vi "clientTCP.vi"(3 "error in":errorcluster, 5 "BrigthField":T1(plugin-control)) -> (0 "error out":errorcluster, 1 "maskCenters":u32[][](array[numeric]), 2 "Segmented":T1(plugin-control))   [LabVIEW 2018]
uses:
  <resource>/objmgr/IMAQImage.rc
panel:
  out "call chain":string[](array[string])
  out "ySize 2":i32
  out "xSize 2":i32
  out "Image 3":T1(plugin-control)
  out "ySize":i32
  out "xSize":i32
  in  "Image File Path":path
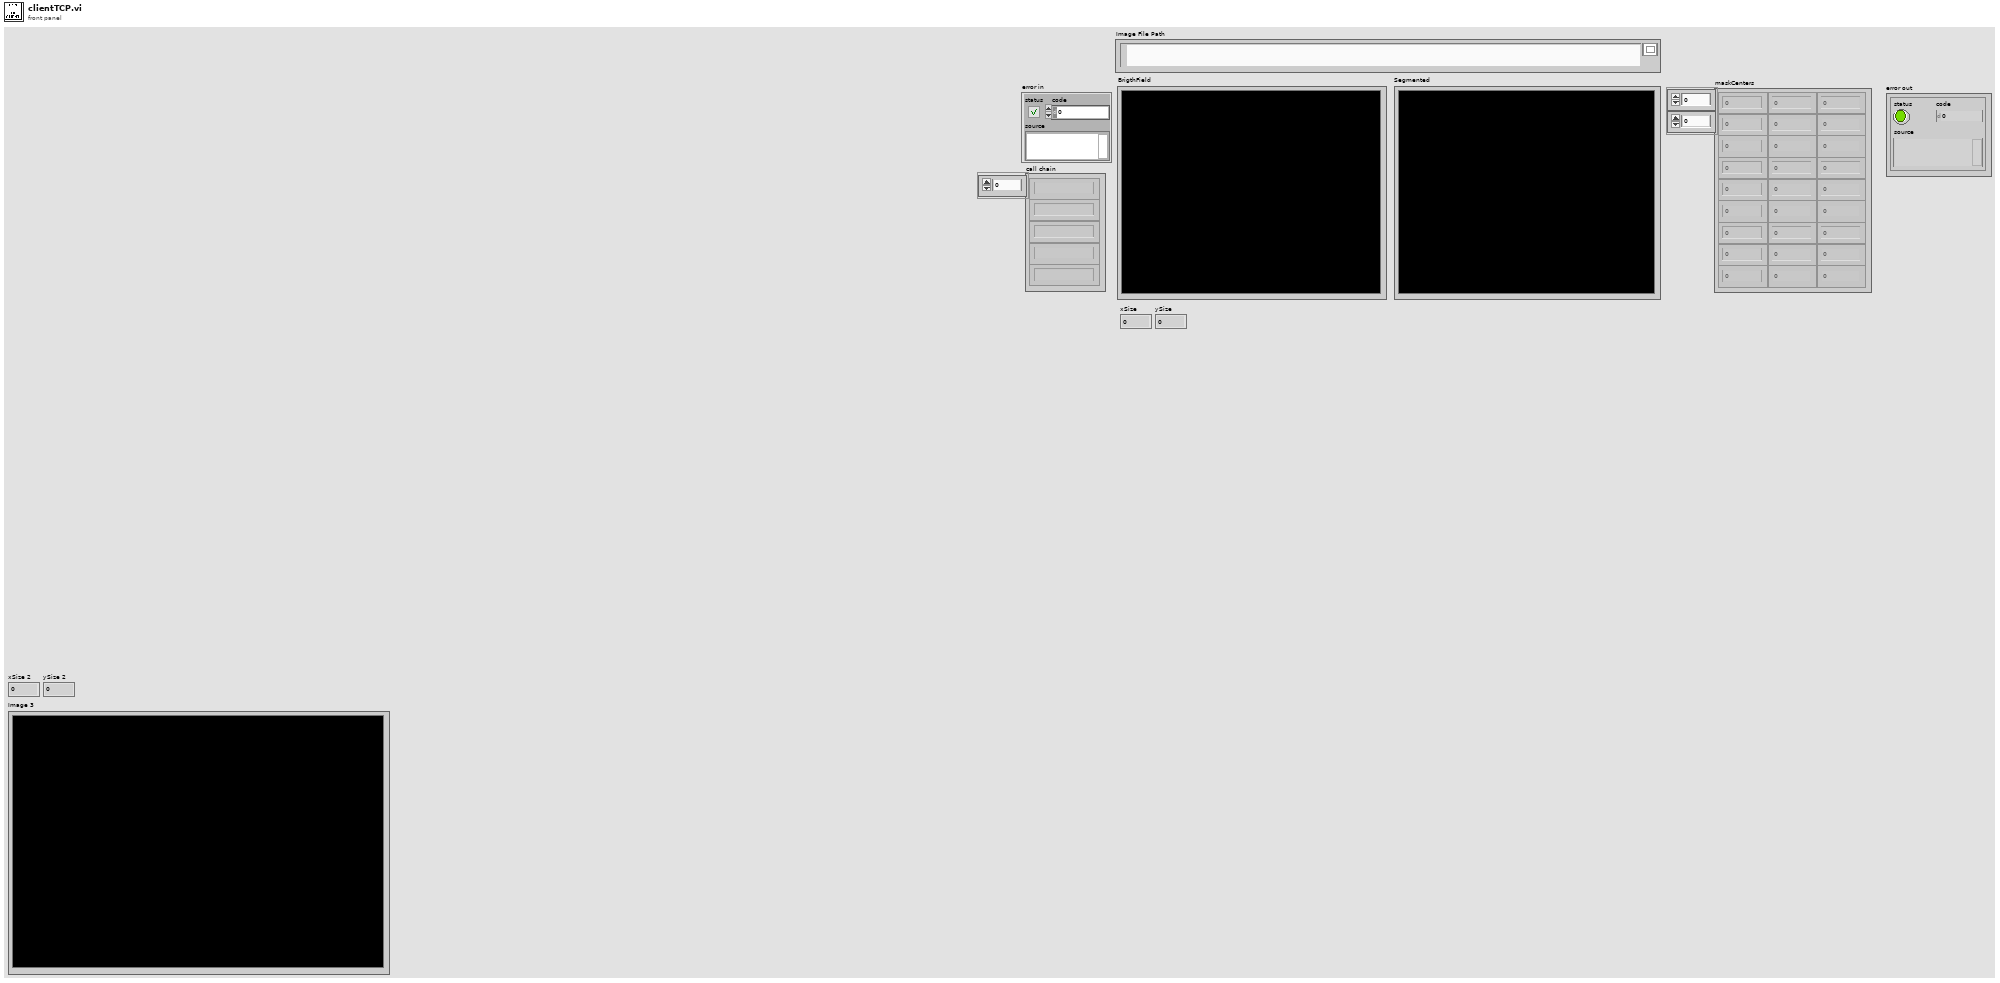
[diagram p1: front panel]
types:
  T1 = typedef "IMAQ Image.ctl" = refnum<image>
  T2 = typedef "Image Type" = u32
  T3 = enum16{"TransferImage", "ReceiveImage", "Disconnect"}
  T4 = enum16{"big-endian, network order", "native, host order", "little-endian"}
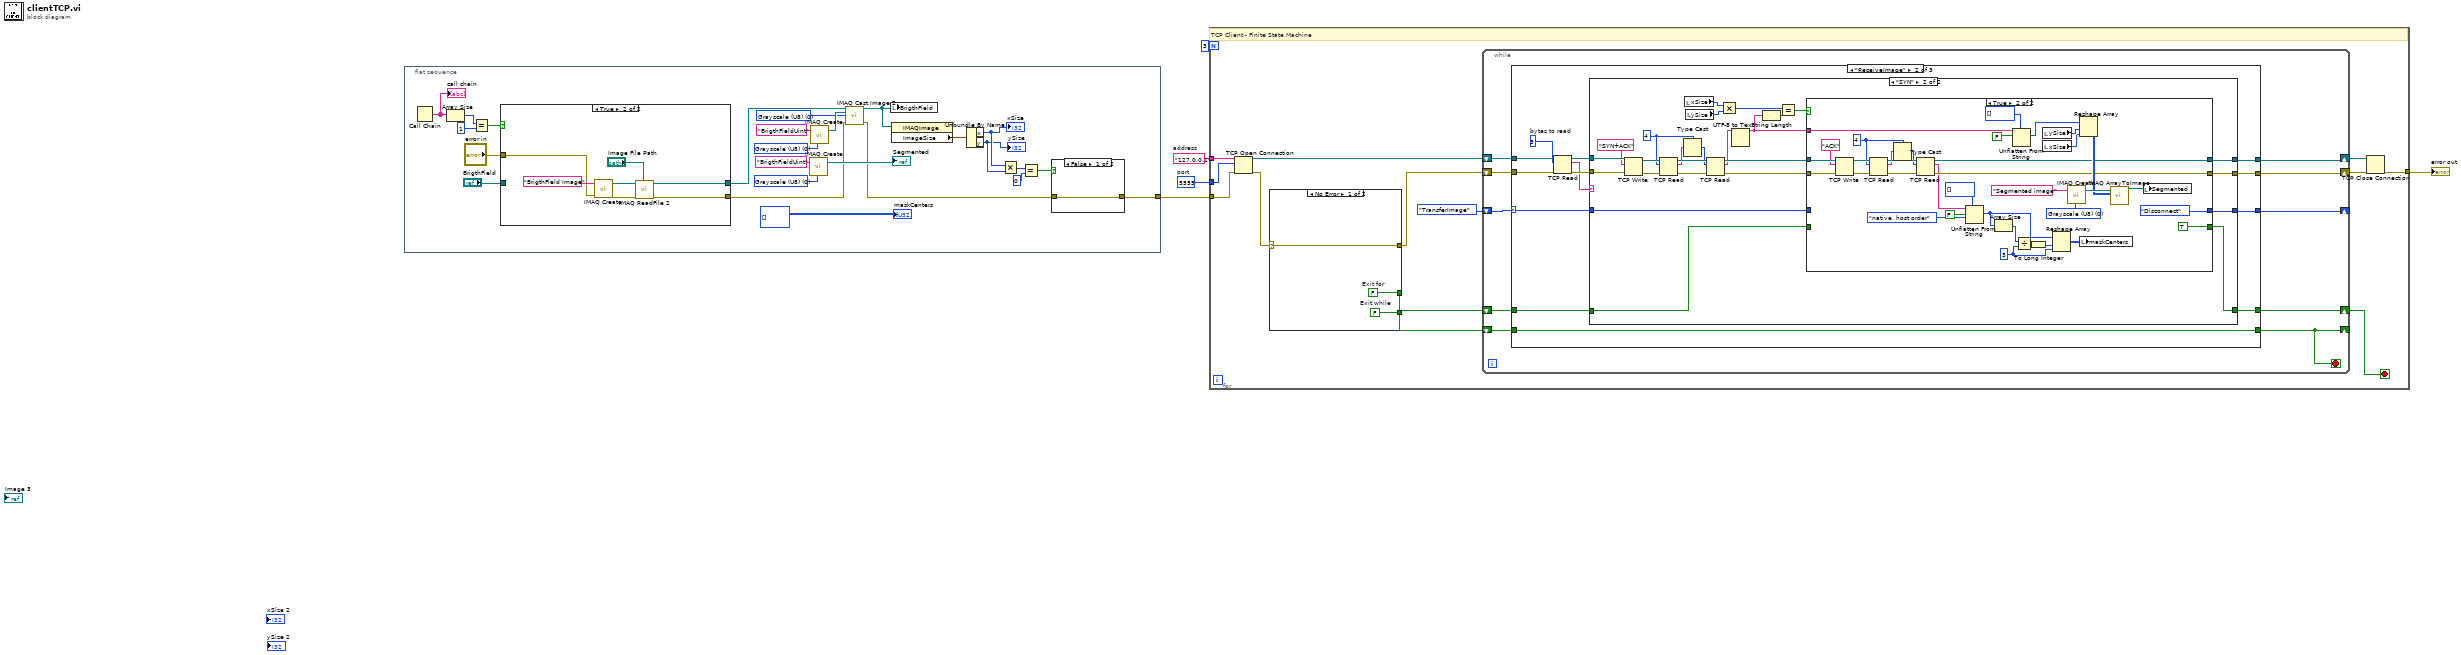
[diagram p0: block diagram]
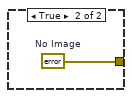
[diagram p2: hidden frame]
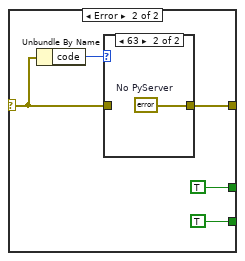
[diagram p4: hidden frame]
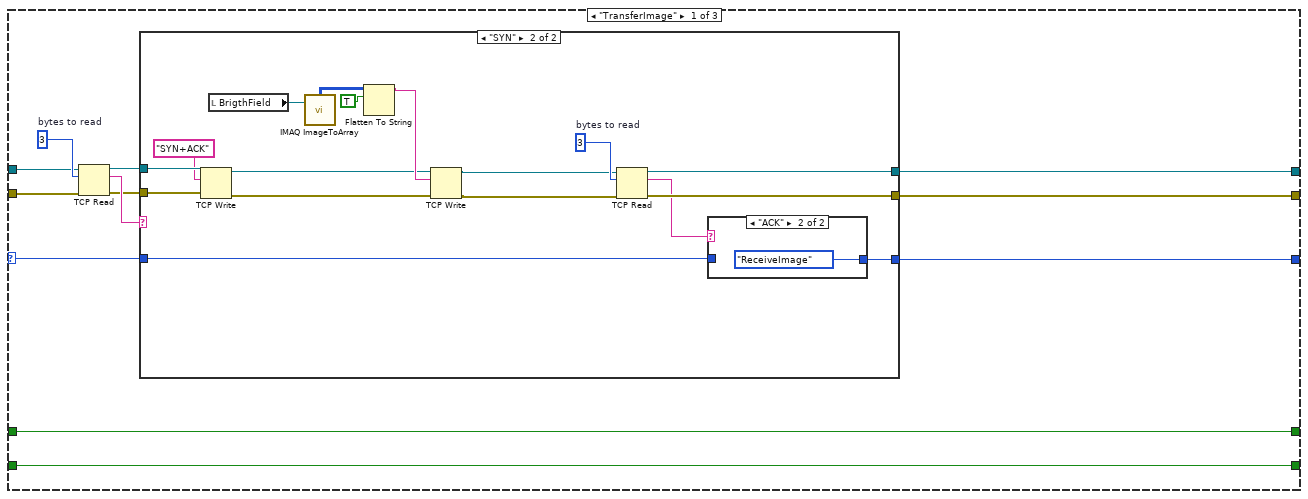
[diagram p6: hidden frame]
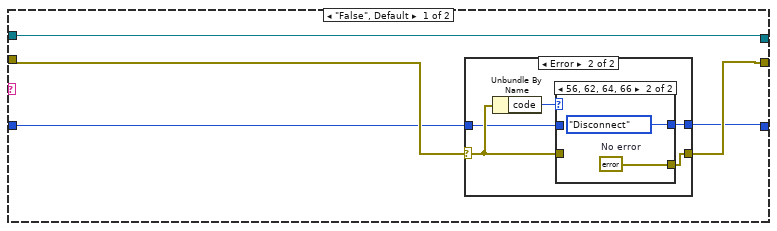
[diagram p7: hidden frame]
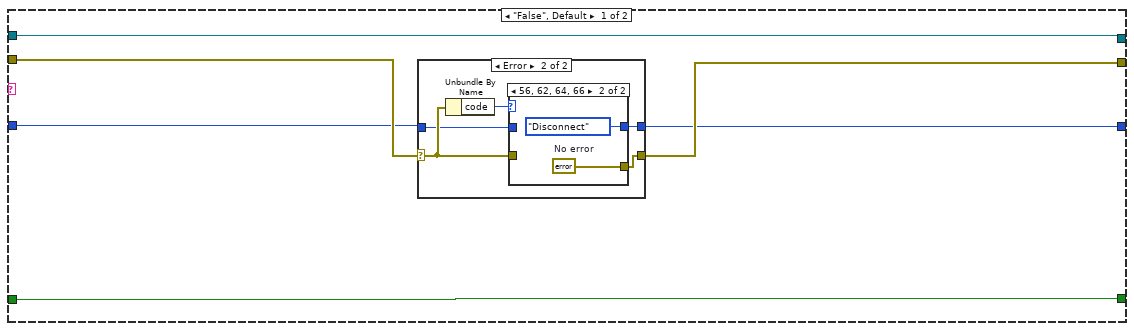
[diagram p11: hidden frame]
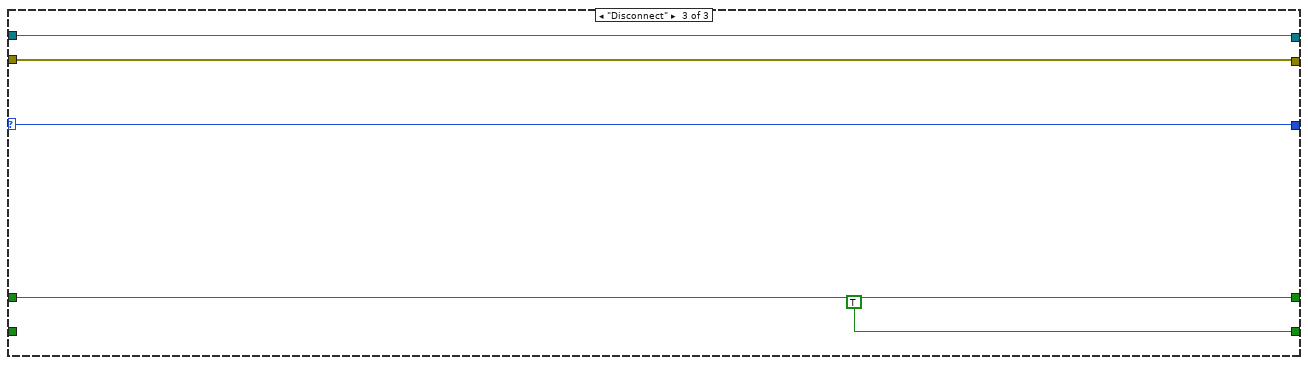
[diagram p15: hidden frame]
diagram:
  w5 = u16 5555  # port
  w4 = "127.0.0.1"  # address
  n1 = flat-sequence {
    tunnel: [w13] -> w2
    frame #0 {
      w20 = T2 0 items=["Grayscale (U8)", "Grayscale (I16)", "Grayscale (SGL)", "Complex (CSG)", "RGB (U32)", "HSL (U32)", "RGB (U64)", "Grayscale (U16)"] ("Image Type")
      w24 = T2 0 items=["Grayscale (U8)", "Grayscale (I16)", "Grayscale (SGL)", "Complex (CSG)", "RGB (U32)", "HSL (U32)", "RGB (U64)", "Grayscale (U16)"] ("Image Type")
      w25 = T2 0 items=["Grayscale (U8)", "Grayscale (I16)", "Grayscale (SGL)", "Complex (CSG)", "RGB (U32)", "HSL (U32)", "RGB (U64)", "Grayscale (U16)"] ("Image Type")
      n2 = Call Chain() -> (call chain=w11:string[])
      "call chain" <- w11
      n3 = Array Size(array=w11) -> (size(s)=w9:i32)
      n4 = Equal?(x=w9, y=1) -> (x = y?=w8:bool)
      n5 = case shown="True" w8 {
        tunnel: [w34 w40] -> w26
        tunnel: "BrigthField" -> [w34 _]
        tunnel: "error in" -> [w33 w37]
        tunnel: [w33 w35] -> w7
        frame False {
        }
        frame True {
          n6 = call "IMAQ Create"("Image Name"="BrigthField Image", "error in (no error)"=w37) -> ("New Image"=w41:T1, "error out"=w36:errorcluster)  [unwired: 3 in]
          n7 = call "IMAQ ReadFile 2"("File Path"="Image File Path", "error in (no error)"=w36, "Image"=w41) -> ("error out"=w35:errorcluster, "Image Out"=w40:T1)  [unwired: 4 in, 3 out]
        }
      }
      n8 = call "IMAQ Create"("Image Name"="BrigthFieldUint", "Image Type"=w24) -> ("New Image"=→"Segmented":T1)  [unwired: 3 in, 1 out]
      n9 = call "IMAQ Create"("Image Name"="BrigthFieldUint", "Image Type"=w25) -> ("New Image"=w27:T1)  [unwired: 3 in, 1 out]
      n10 = call "IMAQ Cast Image 2"("Image Src"=w26, "Image Dst"=w27, "Image Type"=w20, "error in (no error)"=w7) -> ("Image Dst Out"=w19:T1, "error out"=w6:errorcluster)  [unwired: 10 in]
      n11 = local write "BrigthField"(w19) -> ()
      n12 = property class="IMAQImage"(reference=w19) -> ("ImageSize"=w30:cluster{"x":i32, "y":i32})  [unwired: 1 in, 2 out]
      n13 = Unbundle By Name(w30) -> ("x"=w18:i32, "y"=w17:i32)
      "xSize" <- w18
      "ySize" <- w17
      n14 = Multiply(x=w18, y=w17) -> (x*y=w16:i32)
      n15 = Equal?(x=w16, y=0) -> (x = y?=w14:bool)
      n16 = case shown="False" w14 {
        tunnel: w6 -> [w31 _]
        tunnel: [w31 w32] -> w13
        frame False {
        }
        frame True {
          w32 = errorcluster {"status"=TRUE, "code"=101, "source"="No Image"}  # No Image
        }
      }
      "maskCenters" <- u32[][] []
    }
  }
  n17 = for {
    N: 3 -> [_]
    tunnel: w5 -> [w54]
    tunnel: w4 -> [w53]
    tunnel: w2 -> [w47]
    tunnel: [w46] -> w1
    stop <- w48 stop-if-true
    # "TCP Client - Finite State Machine"
    n18 = TCP Open Connection(address=w53, remote port or service name=w54, error in (no error)=w47) -> (connection ID=w51:refnum<k5>, error out=w45:errorcluster)  [unwired: 2 in]
    n19 = case shown="No Error" w45 {
      selector: w45 -> [w57 w61]
      tunnel: [w57 w60] -> w44
      tunnel: [w56 TRUE] -> w43
      tunnel: [w55 TRUE] -> w42
      frame No Error {
        w55 = FALSE  # Exit while
        w56 = FALSE  # Exit for
      }
      frame Error {
        n20 = Unbundle By Name(w61) -> ("code"=w62:i32)
        n21 = case shown="63" w62 {
          tunnel: w61 -> [w63 _]
          tunnel: [w63 w64] -> w60
          frame Default {
          }
          frame 63 {
            w64 = errorcluster {"status"=TRUE, "code"=63, "source"="No PyServer"}  # No PyServer
          }
        }
      }
    }
    n22 = while {
      shift-right: [w69] -> _
      shift-left: T3."TransferImage" -> [w74]
      shift-right: [w71] -> w50
      shift-left: w51 -> [w73]
      shift-right: [w70] -> w49
      shift-left: w44 -> [w72]
      shift-right: [w67] -> _
      shift-left: w42 -> [w68]
      shift-right: [w66] -> w48
      shift-left: w43 -> [w65]
      stop <- w67 stop-if-true
      n23 = case shown="\"ReceiveImage\"" w74 {
        selector: w74 -> [w77 w127 w218]
        tunnel: w73 -> [w85 w126 w220]
        tunnel: w72 -> [w84 w125 w219]
        tunnel: [w80 w130 w220] -> w71
        tunnel: [w79 w129 w219] -> w70
        tunnel: [w78 w128 w218] -> w69
        tunnel: [w76 w124 TRUE] -> w67
        tunnel: w68 -> [w76 w124 _]
        tunnel: [w75 w123 w216] -> w66
        tunnel: w65 -> [w75 w122 w216]
        frame "TransferImage" {
          w86 = 3  # bytes to read
          n24 = TCP Read(connection ID=w85, bytes to read=w86, error in (no error)=w84) -> (connection ID out=w82:refnum<k5>, data out=w83:string, error out=w81:errorcluster)  [unwired: 2 in]
          n25 = case shown="\"SYN\"" w83 {
            tunnel: w82 -> [w91 w119]
            tunnel: w81 -> [w90 w118]
            tunnel: [w91 w112] -> w80
            tunnel: [w89 w111] -> w79
            tunnel: [w88 w109] -> w78
            tunnel: w77 -> [w87 w108]
            frame "False", Default {
              n26 = case shown="Error" w90 {
                selector: w90 -> [w93 w97]
                tunnel: [w93 w96] -> w89
                tunnel: [w92 w95] -> w88
                tunnel: w87 -> [w92 w94]
                frame No Error {
                }
                frame Error {
                  n27 = Unbundle By Name(w97) -> ("code"=w98:i32)
                  n28 = case shown="56, 62, 64, 66" w98 {
                    tunnel: w97 -> [w100 _]
                    tunnel: [w100 w102] -> w96
                    tunnel: [w99 T3."Disconnect"] -> w95
                    tunnel: w94 -> [w99 _]
                    frame Default {
                    }
                    frame 56, 62, 64, 66 {
                      w102 = errorcluster {"status"=FALSE, "code"=0, "source"=""}  # No error
                    }
                  }
                }
              }
            }
            frame "SYN" {
              w115 = 3  # bytes to read
              n29 = TCP Write(connection ID=w119, data in="SYN+ACK", error in (no error)=w118) -> (connection ID out=w104:refnum<k5>, error out=w103:errorcluster)  [unwired: 2 out]
              n30 = local read "BrigthField"() -> (w116:T1)
              n31 = call "IMAQ ImageToArray"("Image"=w116) -> ("Image Pixels (U8)"=w107:u8[][])  [unwired: 3 in, 4 out]
              n32 = Flatten To String(anything=w107, prepend array or string size? (T)=TRUE) -> (data string=w106:string)  [unwired: 2 in, 2 out]
              n33 = TCP Write(connection ID=w104, data in=w106, error in (no error)=w103) -> (connection ID out=w114:refnum<k5>, error out=w113:errorcluster)  [unwired: 2 out]
              n34 = TCP Read(connection ID=w114, bytes to read=w115, error in (no error)=w113) -> (connection ID out=w112:refnum<k5>, data out=w110:string, error out=w111:errorcluster)  [unwired: 2 in]
              n35 = case shown="\"ACK\"" w110 {
                tunnel: [w120 T3."ReceiveImage"] -> w109
                tunnel: w108 -> [w120 _]
                frame "False", Default {
                }
                frame "ACK" {
                }
              }
            }
          }
        }
        frame "ReceiveImage" {
          w131 = 3  # bytes to read
          n36 = TCP Read(connection ID=w126, bytes to read=w131, error in (no error)=w125) -> (connection ID out=w133:refnum<k5>, data out=w132:string, error out=w134:errorcluster)  [unwired: 2 in]
          n37 = case shown="\"SYN\"" w132 {
            tunnel: w133 -> [w140 w176]
            tunnel: w134 -> [w138 w175]
            tunnel: [w140 w169] -> w130
            tunnel: [w137 w168] -> w129
            tunnel: [w135 w166] -> w128
            tunnel: w127 -> [w136 w165]
            tunnel: [w139 w163] -> w123
            tunnel: w122 -> [w139 w162]
            frame "False", Default {
              n38 = case shown="Error" w138 {
                selector: w138 -> [w142 w146]
                tunnel: [w142 w145] -> w137
                tunnel: [w141 w144] -> w135
                tunnel: w136 -> [w141 w143]
                frame No Error {
                }
                frame Error {
                  n39 = Unbundle By Name(w146) -> ("code"=w147:i32)
                  n40 = case shown="56, 62, 64, 66" w147 {
                    tunnel: w146 -> [w149 _]
                    tunnel: [w149 w151] -> w145
                    tunnel: [w148 T3."Disconnect"] -> w144
                    tunnel: w143 -> [w148 _]
                    frame Default {
                    }
                    frame 56, 62, 64, 66 {
                      w151 = errorcluster {"status"=FALSE, "code"=0, "source"=""}  # No error
                    }
                  }
                }
              }
            }
            frame "SYN" {
              w152 = 4
              n41 = TCP Write(connection ID=w176, data in="SYN+ACK", error in (no error)=w175) -> (connection ID out=w158:refnum<k5>, error out=w156:errorcluster)  [unwired: 2 out]
              n42 = TCP Read(connection ID=w158, bytes to read=w152, error in (no error)=w156) -> (connection ID out=w157:refnum<k5>, data out=w154:string, error out=w155:errorcluster)  [unwired: 2 in]
              n43 = Type Cast(type=w152, x=w154) -> (*(type *) &x=w153:i32)
              n44 = local read "xSize"() -> (w172:i32)
              n45 = local read "ySize"() -> (w173:i32)
              n46 = TCP Read(connection ID=w157, bytes to read=w153, error in (no error)=w155) -> (connection ID out=w170:refnum<k5>, data out=w164:string, error out=w167:errorcluster)  [unwired: 2 in]
              n47 = Multiply(x=w172, y=w173) -> (x*y=w161:i32)
              n48 = UTF-8 to Text(11:w164) -> (3:w160:string)  [unwired: 2 in, 1 out]
              n49 = String Length(string=w160) -> (length=w159:i32)
              n50 = Equal?(x=w161, y=w159) -> (x = y?=w171:bool)
              n51 = case shown="True" w171 {
                tunnel: w160 -> [_ w214]
                tunnel: w170 -> [w180 w204]
                tunnel: [w180 w198] -> w169
                tunnel: [w179 w196] -> w168
                tunnel: w167 -> [w179 w203]
                tunnel: [w178 T3."Disconnect"] -> w166
                tunnel: w165 -> [w178 _]
                tunnel: [w177 TRUE] -> w163
                tunnel: w162 -> [w177 _]
                frame False {
                }
                frame True {
                  w181 = T2 0 items=["Grayscale (U8)", "Grayscale (I16)", "Grayscale (SGL)", "Complex (CSG)", "RGB (U32)", "HSL (U32)", "RGB (U64)", "Grayscale (U16)"] ("Image Type")
                  w184 = 3 ("dimension size")
                  w194 = 4
                  n52 = TCP Write(connection ID=w204, data in="ACK", error in (no error)=w203) -> (connection ID out=w197:refnum<k5>, error out=w195:errorcluster)  [unwired: 2 out]
                  n53 = TCP Read(connection ID=w197, bytes to read=w194, error in (no error)=w195) -> (connection ID out=w201:refnum<k5>, data out=w199:string, error out=w200:errorcluster)  [unwired: 2 in]
                  n54 = Type Cast(type=w194, x=w199) -> (*(type *) &x=w192:i32)
                  n55 = TCP Read(connection ID=w201, bytes to read=w192, error in (no error)=w200) -> (connection ID out=w198:refnum<k5>, data out=w188:string, error out=w196:errorcluster)  [unwired: 2 in]
                  n56 = Unflatten From String(type=u32[] [] ("Image Pixels (U8)"), binary string=w188, data includes array or string size? (T)=FALSE, byte order (0:big-endian, network order)=T4."native, host order") -> (value=w186:u32[])  [unwired: 1 in, 2 out]
                  n57 = Array Size(array=w186) -> (size(s)=w185:i32)
                  n58 = Unflatten From String(type=u8[] [] ("Image Pixels (U8)"), binary string=w214, data includes array or string size? (T)=FALSE) -> (value=w213:u8[])  [unwired: 2 in, 2 out]
                  n59 = Divide(x=w185, y=w184) -> (x/y=w191:dbl)
                  n60 = To Long Integer(number=w191) -> (32bit integer=w190:i32)
                  n61 = local read "ySize"() -> (w212:i32)
                  n62 = local read "xSize"() -> (w211:i32)
                  n63 = Reshape Array(w186, w190, w184) -> (w182:u32[][])
                  n64 = call "IMAQ Create"("Image Name"="Segmented image", "Image Type"=w181) -> ("New Image"=w209:T1)  [unwired: 3 in, 1 out]
                  n65 = Reshape Array(w213, w212, w211) -> (w208:u8[][])
                  n66 = local write "maskCenters"(w182) -> ()
                  n67 = call "IMAQ ArrayToImage"("Image Pixels (U8)"=w208, "Image"=w209) -> ("Image Out"=w207:T1)  [unwired: 8 in, 1 out]
                  n68 = local write "Segmented"(w207) -> ()
                }
              }
            }
          }
        }
        frame "Disconnect" {
        }
      }
    }
    n69 = TCP Close Connection(connection ID=w50, error in (no error)=w49) -> (error out=w46:errorcluster)  [unwired: 1 in, 1 out]
  }
  "error out" <- w1
